vi "CIF File Location.vi"(11 "LocationType":T1) -> (3 "Location":path)   [LabVIEW 2021, in "CIF Configuration File.lvlib"]
uses:
  CIF Configuration File.lvlib
  typedef/Location Type.ctl
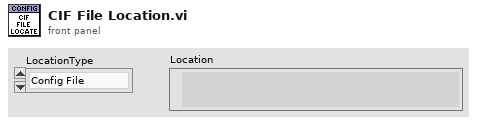
[diagram p1: front panel]
types:
  T1 = typedef "CIF Configuration File.lvlib/Location Type.ctl" = enum16{"Config File", "Manager", "Protos", "Plugins", "UI Plugins", "Logs", "Orchestrations"}
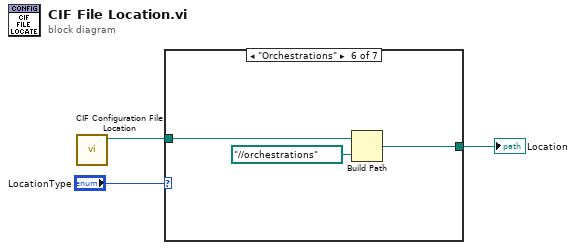
[diagram p0: block diagram]
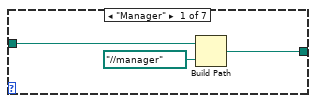
[diagram p2: hidden frame]
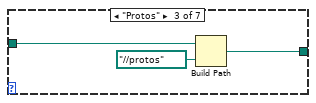
[diagram p4: hidden frame]
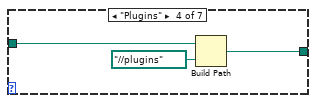
[diagram p5: hidden frame]
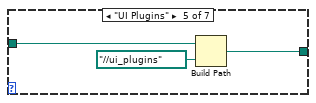
[diagram p6: hidden frame]
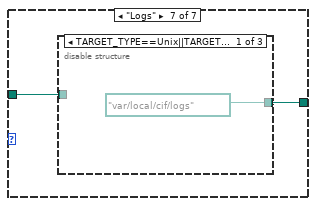
[diagram p7: hidden frame]
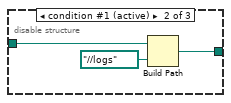
[diagram p8: hidden frame]
diagram:
  n1 = call "CIF Configuration File Location.vi"() -> ("configuration file path"=w2:path)  [unwired: 11 in]
  n2 = case shown="\"Orchestrations\"" "LocationType" {
    tunnel: w2 -> [w6 w7 w10 w13 w16 w19 w20]
    tunnel: [w4 w7 w8 w11 w14 w17 w21] -> w1
    frame "Manager" {
      n3 = Build Path(base path=w6, name or relative path=path "../../manager") -> (appended path=w4:path)
    }
    frame "Config File" {
    }
    frame "Protos" {
      n4 = Build Path(base path=w10, name or relative path=path "../../protos") -> (appended path=w8:path)
    }
    frame "Plugins" {
      n5 = Build Path(base path=w13, name or relative path=path "../../plugins") -> (appended path=w11:path)
    }
    frame "UI Plugins" {
      n6 = Build Path(base path=w16, name or relative path=path "../../ui_plugins") -> (appended path=w14:path)
    }
    frame "Orchestrations" {
      n7 = Build Path(base path=w19, name or relative path=path "../../orchestrations") -> (appended path=w17:path)
    }
    frame "Logs" {
      n8 = disable-structure shown="TARGET_TYPE==Unix||TARGET_TYPE==RT" {
        disable-tunnel: [path "/var/local/cif/logs" ("configuration file path") w24 _] -> w21
        disable-tunnel: w20 -> [_ w23 _]
        frame condition #0 {
        }
        frame condition #1 (active) {
          n9 = Build Path(base path=w23, name or relative path=path "../../logs") -> (appended path=w24:path)
        }
        frame condition #2 {
        }
      }
    }
  }
  "Location" <- w1
